vi "libTSMaster_DLL.vi"() -> ()   [LabVIEW 2014]
panel:
  in  "libTSMaster_DLL":path
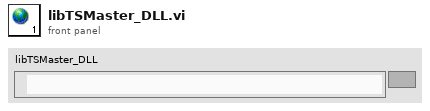
[diagram p1: front panel]
diagram:
